vi "Auto Vision.vi"(11 "Run?":bool) -> (2 "Side?":dbl, 3 "Done":bool)   [LabVIEW 2013]
panel:
  out "element":dbl
  out "Particle Measurements (Pixels)":dbl[][](array[numeric]) format="%.2f"
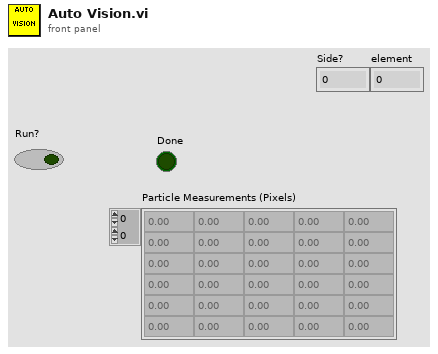
[diagram p1: front panel]
types:
  T1 = typedef "WPI_CameraDevRef.ctl" = cluster{"Camera Address":string, "CameraStatus":errorcluster, "Acquire Image Notifier":refnum<notifier>}
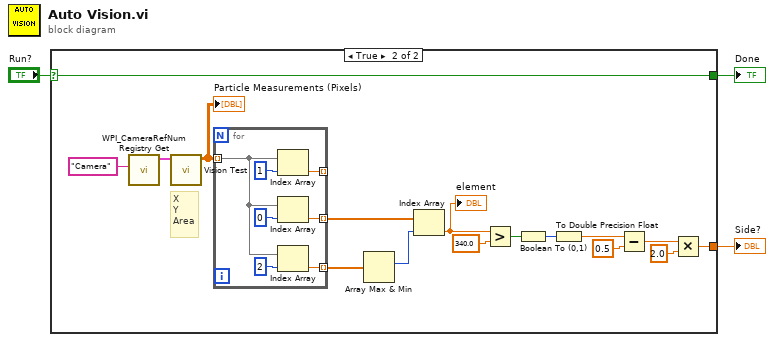
[diagram p0: block diagram]
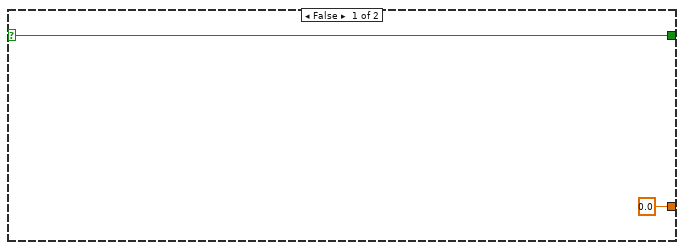
[diagram p2: hidden frame]
diagram:
  n1 = case shown="True" "Run?" {
    selector: "Run?" -> [w5 w21]
    tunnel: [w5 w21] -> w2
    tunnel: [0.0 w12] -> w1
    frame False {
    }
    frame True {
      # "X\nY\nArea"
      n2 = call <vilib>:"WPI_CameraRefNum Registry Get.vi"("refnum name"="Camera") -> ("CameraDevRef"=w19:T1)  [unwired: 9 in, 1 out]
      n3 = call "Vision Test.vi"("CameraDevRef"=w19) -> ("Particle Measurements (Pixels)"=w20:dbl[][])  [unwired: 9 in, 1 out]
      "Particle Measurements (Pixels)" <- w20
      n4 = for {
        tunnel: w20 -> [w23] mode=indexing
        tunnel: [w26] -> w10 mode=indexing
        tunnel: [w25] -> _ mode=indexing
        tunnel: [w22] -> w11 mode=indexing
        n5 = Index Array(array=w23, index=1) -> (element=w25:dbl)
        n6 = Index Array(array=w23, index=0) -> (element=w26:dbl)
        n7 = Index Array(array=w23, index=2) -> (element=w22:dbl)
      }
      n8 = Array Max & Min(array=w11) -> (max index (indices)=w9:i32)  [unwired: 3 out]
      n9 = Index Array(array=w10, index=w9) -> (element=w6:dbl)
      "element" <- w6
      n10 = Greater?(x=w6, y=340.0) -> (0:w7:bool)
      n11 = Boolean To (0,1)(Boolean=w7) -> (0, 1=w13:i16)
      n12 = To Double Precision Float(number=w13) -> (double precision float=w14:dbl)
      n13 = Subtract(x=w14, y=0.5) -> (x-y=w16:dbl)
      n14 = Multiply(x=w16, y=2.0) -> (x*y=w12:dbl)
    }
  }
  "Done" <- w2
  "Side?" <- w1
